vi "C_A_code.vi"(1 "NKA id":dbl=1.0, 2 "Delay":dbl) -> (0 "Value":i32[](array[numeric]))   [LabVIEW 2020]
uses:
  <vilib>/Enthought/Python Integration Toolkit/api/Unpack Int Array.vi
  <vilib>/Enthought/Python Integration Toolkit/Python Integration Toolkit.lvlib
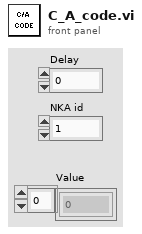
[diagram p1: front panel]
types:
  T1 = typedef "Python Integration Toolkit.lvlib/Session ID.ctl" = u64
  T2 = typedef "Python Integration Toolkit.lvlib/Python Objects.ctl" = variant
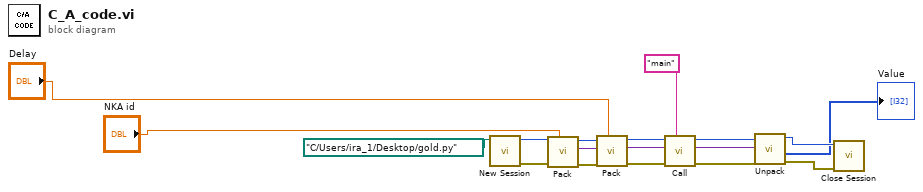
[diagram p0: block diagram]
diagram:
  n1 = call <vilib>:"New Session.vi"("Path to Python Module (.py File)"=path "C:/Users/ira_1/Desktop/gold.py") -> ("error out"=w6:errorcluster, "Session ID out"=w7:T1)  [unwired: 9 in]
  n2 = call <vilib>:"Pack.vi"("Argument"="NKA id", "error in (no error)"=w6, "Session ID"=w7) -> ("error out"=w5:errorcluster, "Python Object References Out"=w3:T2, "Session ID out"=w4:T1)  [unwired: 6 in]
  n3 = call <vilib>:"Pack.vi"("Argument"="Delay", "error in (no error)"=w5, "Python Object References In"=w3, "Session ID"=w4) -> ("error out"=w12:errorcluster, "Python Object References Out"=w9:T2, "Session ID out"=w18:T1)  [unwired: 5 in]
  n4 = call <vilib>:"Call.vi"("Function or Method Name"="main", "error in (no error)"=w12, "Python Object References In"=w9, "Session ID"=w18) -> ("error out"=w13:errorcluster, "Python Object References Out"=w14:T2, "Session ID out"=w17:T1)  [unwired: 5 in]
  n5 = call-poly <vilib>:"Unpack.vi"("error in (no error)"=w13, "Python Object References In"=w14, "Session ID"=w17) -> ("error out"=w15:errorcluster, "Value"=→"Value":i32[], "Session ID out"=w16:T1)  [unwired: 5 in, 1 out]
  n6 = call <vilib>:"Close Session.vi"("error in (no error)"=w15, "Session ID"=w16) -> ()  [unwired: 9 in, 1 out]
